vi "FGV Stoermeldungsdatei.vi"(6 "Aktionen":T1, 8 "Fehler (Eingang, kein Fehler)":errorcluster, 11 "Neue Tabelle":string[][](array[string])) -> (0 "Fehler (Ausgang)":errorcluster, 1 "abschaltend":bool[](array[boolean]), 2 "quittieren?":bool[](array[boolean]), 3 "Ansprechverzögerung":dbl[](array[numeric]), 4 "Text":string[](array[string]), 5 "max Nummer":i32)   [LabVIEW 2020, in "Stoerungen.lvlib"]
uses:
  Stoerungen.lvlib
  FGV Stoerungsdatei Aktionen.ctl
  Sprachverwaltung/FGV Aktion Tabelle zerlegen.ctl
  Allgemein/allgemeine Sub-VIs.lvlib
  Sprachverwaltung/Sprachverwaltung.lvlib
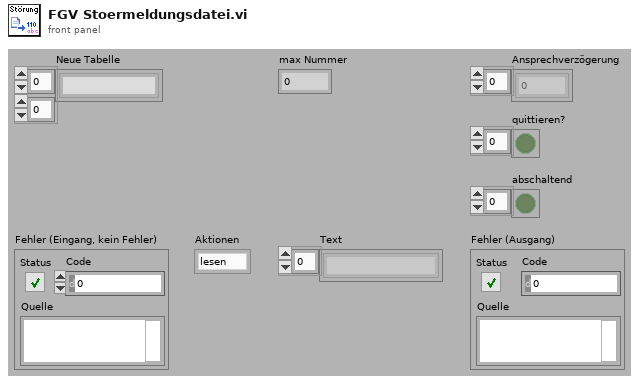
[diagram p1: front panel]
types:
  T1 = typedef "Stoerungen.lvlib/FGV Stoerungsdatei Aktionen.ctl" = enum16{"lesen", "laden", "Neue Werte"}
  T2 = typedef "Sprachverwaltung.lvlib/FGV Aktion Tabelle zerlegen.ctl" = enum16{"laden", "vereinzeln", "speichern"}
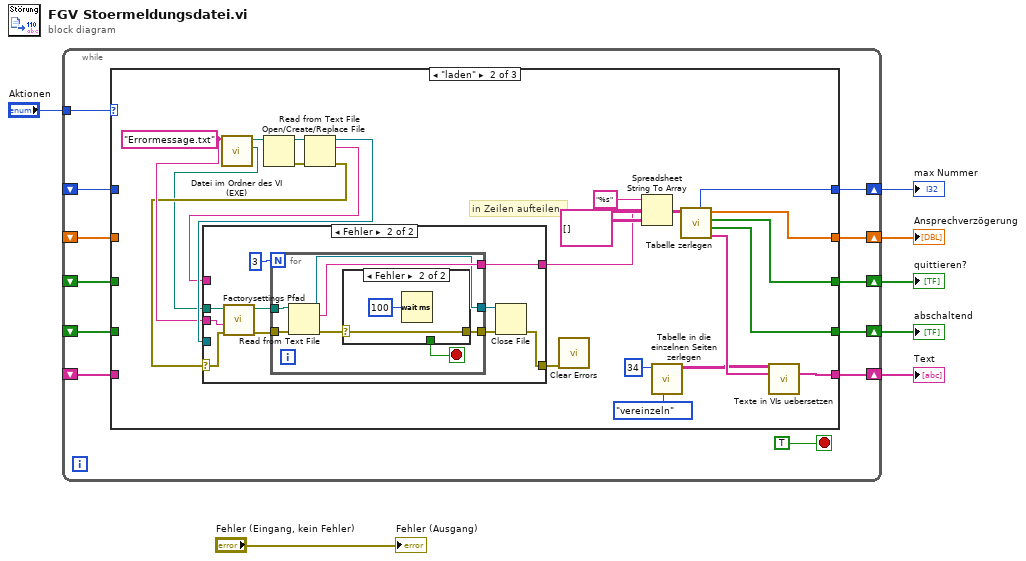
[diagram p0: block diagram]
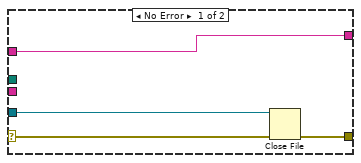
[diagram p3: hidden frame]
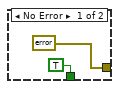
[diagram p4: hidden frame]
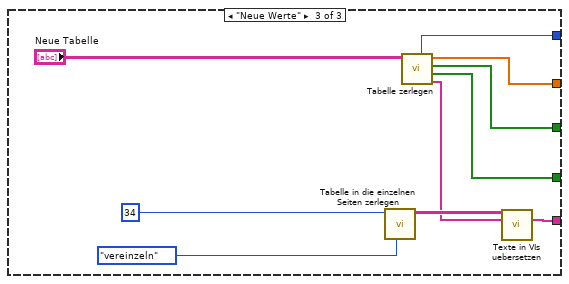
[diagram p5: hidden frame]
diagram:
  n1 = while {
    shift-right: [w17] -> w6
    shift-left: _ -> [w8]
    shift-right: [w16] -> w5
    shift-left: _ -> [w9]
    shift-right: [w15] -> w4
    shift-left: _ -> [w10]
    shift-right: [w14] -> w3
    shift-left: _ -> [w11]
    shift-right: [w13] -> w2
    shift-left: _ -> [w12]
    tunnel: "Aktionen" -> [w18]
    stop <- TRUE stop-if-true
    n2 = case shown="\"laden\"" w18 {
      tunnel: [w24 w43 w81] -> w17
      tunnel: [w23 w40 w78] -> w16
      tunnel: [w22 w41 w79] -> w15
      tunnel: [w21 w42 w80] -> w14
      tunnel: [w20 w38 w73] -> w13
      tunnel: w12 -> [w20 _ _]
      tunnel: w11 -> [w21 _ _]
      tunnel: w10 -> [w22 _ _]
      tunnel: w9 -> [w23 _ _]
      tunnel: w8 -> [w24 _ _]
      frame "lesen", Default {
      }
      frame "laden" {
        w33 = "Errormessage.txt" ("Dateiname")
        # "in Zeilen aufteilen"
        n3 = call "Datei im Ordner des VI (EXE).vi"("Dateiname"=w33) -> ("Ordner des Haupt-VIs"=w28:path, "Dateipfad im Ordner des Haupt-VIs"=w25:path)  [unwired: 8 in, 1 out]
        n4 = Open/Create/Replace File(file path (use dialog)=w25) -> (refnum out=w26:refnum<file>, error out=w27:errorcluster)  [unwired: 5 in, 1 out]
        n5 = Read from Text File(file (use dialog)=w26, error in=w27) -> (refnum out=w34:refnum<file>, text=w32:string, error out=w29:errorcluster)  [unwired: 3 out]
        n6 = case shown="Fehler" w29 {
          selector: w29 -> [w49 w51]
          tunnel: w28 -> [_ w53]
          tunnel: w32 -> [w50 _]
          tunnel: [w50 w59] -> w31
          tunnel: [w47 w57] -> w30
          tunnel: w34 -> [w48 _]
          tunnel: w33 -> [_ w52]
          frame No Error {
            n7 = Close File(refnum=w48, error in=w49) -> (error out=w47:errorcluster)  [unwired: 1 out]
          }
          frame Error {
            n8 = call "Factorysettings Pfad.vi"("error in (no error)"=w51, "Dateiname"=w52, "Ordner des Haupt-VIs"=w53) -> ("error out"=w54:errorcluster, "Pfad Factorysettings"=w55:path)  [unwired: 7 in]
            n9 = for {
              N: 3 -> [_]
              tunnel: w54 -> [w65]
              tunnel: w55 -> [w64]
              tunnel: [w63] -> w59
              tunnel: [w62] -> w58
              tunnel: [w61] -> w56
              stop <- w66 stop-if-true
              n10 = Read from Text File(file (use dialog)=w64, error in=w65) -> (refnum out=w61:refnum<file>, text=w63:string, error out=w67:errorcluster)  [unwired: 2 in, 1 out]
              n11 = case shown="Fehler" w67 {
                selector: w67 -> [_ w70]
                tunnel: [TRUE _] -> w66
                tunnel: [errorcluster {"status"=FALSE, "code"=0, "source"=""} ("error IO") w70] -> w62
                frame No Error {
                }
                frame Error {
                  n12 = Wait (ms)(milliseconds to wait=u32 100 ("Zu wartende ms")) -> ()  [unwired: 1 out]
                }
              }
            }
            n13 = Close File(refnum=w56, error in=w58) -> (error out=w57:errorcluster)  [unwired: 1 out]
          }
        }
        n14 = call <vilib>:"Clear Errors.vi"("error in (no error)"=w30) -> ()  [unwired: 5 in, 2 out]
        n15 = Spreadsheet String To Array(format string="%s" ("Format-String"), spreadsheet string=w31, array type (2D Dbl)=string[][] []) -> (array=w44:string[][])  [unwired: 1 out]
        n16 = call "Tabelle in die einzelnen Seiten zerlegen.vi"("Aktion"=FGV_Aktion_Tabelle_zerlegen."vereinzeln", "Index (Seite)"=34) -> ("Sprachliste"=w36:string[][])  [unwired: 7 in, 2 out]
        n17 = call "Tabelle zerlegen.vi"("Tabelle"=w44) -> ("Text"=w39:string[], "abschaltend"=w42:bool[], "quittieren?"=w41:bool[], "Ansprechverzögerung"=w40:dbl[], "max Nummer"=w43:i32)  [unwired: 6 in]
        n18 = call "Texte in VIs uebersetzen.vi"("Sprachliste"=w36, "String-Array zum Übersetzen"=w39) -> ("String-Array zum Übersetzen"=w38:string[])  [unwired: 9 in, 4 out]
      }
      frame "Neue Werte" {
        n19 = call "Tabelle in die einzelnen Seiten zerlegen.vi"("Aktion"=FGV_Aktion_Tabelle_zerlegen."vereinzeln", "Index (Seite)"=34) -> ("Sprachliste"=w75:string[][])  [unwired: 7 in, 2 out]
        n20 = call "Tabelle zerlegen.vi"("Tabelle"="Neue Tabelle") -> ("Text"=w74:string[], "abschaltend"=w80:bool[], "quittieren?"=w79:bool[], "Ansprechverzögerung"=w78:dbl[], "max Nummer"=w81:i32)  [unwired: 6 in]
        n21 = call "Texte in VIs uebersetzen.vi"("Sprachliste"=w75, "String-Array zum Übersetzen"=w74) -> ("String-Array zum Übersetzen"=w73:string[])  [unwired: 9 in, 4 out]
      }
    }
  }
  "max Nummer" <- w6
  "Ansprechverzögerung" <- w5
  "quittieren?" <- w4
  "abschaltend" <- w3
  "Text" <- w2
  "Fehler (Ausgang)" <- "Fehler (Eingang, kein Fehler)"
